vi "SetVariable.vi"(7 "VISA resource name":refnum<visa-resource-name>, 8 "error in (no error)":errorcluster, 9 "Vaste käsk":string="E", 10 "Sisu":string, 11 "Käsk":string="F") -> (3 "Väljund":string)   [LabVIEW 2012]
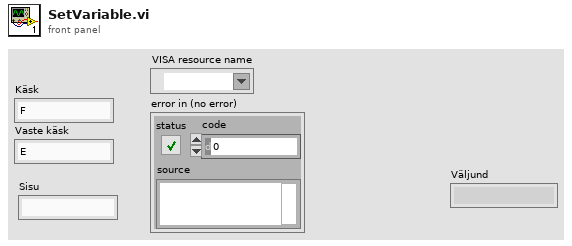
[diagram p1: front panel]
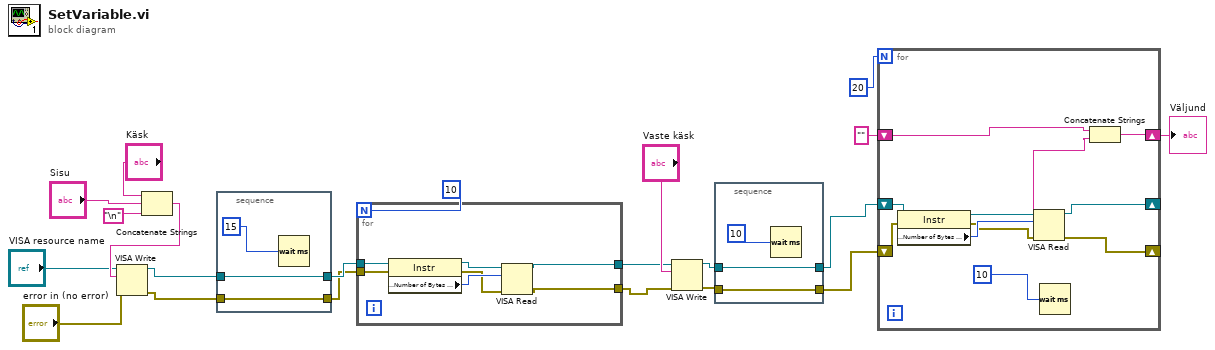
[diagram p0: block diagram]
diagram:
  n1 = Concatenate Strings("Käsk", "Sisu", "\n") -> (w16:string)
  n2 = VISA Write(VISA resource name="VISA resource name", write buffer=w16, error in (no error)="error in (no error)") -> (VISA resource name out=w21:refnum<visa-resource-name>, error out=w20:errorcluster)  [unwired: 1 out]
  n3 = stacked-sequence {
    tunnel: w20 -> [w24]
    tunnel: [w24] -> w18
    tunnel: w21 -> [w23]
    tunnel: [w23] -> w19
    frame #0 {
      n4 = Wait (ms)(milliseconds to wait=u32 15 ("delay Command")) -> ()  [unwired: 1 out]
    }
  }
  n5 = for {
    N: 10 -> [_]
    tunnel: w19 -> [w31]
    tunnel: w18 -> [w30]
    tunnel: [w26] -> w9
    tunnel: [w25] -> w8
    n6 = property class="Instr"(reference=w31, error in=w30) -> (reference out=w29:refnum<visa-resource-name>, error out=w27:errorcluster, "Serial Settings:Number of Bytes at Serial Port"=w28:u32)
    n7 = VISA Read(VISA resource name=w29, byte count=w28, error in (no error)=w27) -> (VISA resource name out=w26:refnum<visa-resource-name>, error out=w25:errorcluster)  [unwired: 2 out]
  }
  n8 = VISA Write(VISA resource name=w9, write buffer="Vaste käsk", error in (no error)=w8) -> (VISA resource name out=w11:refnum<visa-resource-name>, error out=w10:errorcluster)  [unwired: 1 out]
  n9 = stacked-sequence {
    tunnel: w10 -> [w34]
    tunnel: [w34] -> w7
    tunnel: w11 -> [w33]
    tunnel: [w33] -> w6
    frame #0 {
      n10 = Wait (ms)(milliseconds to wait=u32 10 ("delay Input")) -> ()  [unwired: 1 out]
    }
  }
  n11 = for {
    N: 20 -> [_]
    shift-right: [w35] -> w3
    shift-left: "" -> [w36]
    shift-right: [w40] -> _
    shift-left: w6 -> [w38]
    shift-right: [w39] -> _
    shift-left: w7 -> [w41]
    n12 = property class="Instr"(reference=w38, error in=w41) -> (reference out=w45:refnum<visa-resource-name>, error out=w43:errorcluster, "Serial Settings:Number of Bytes at Serial Port"=w44:u32)
    n13 = VISA Read(VISA resource name=w45, byte count=w44, error in (no error)=w43) -> (VISA resource name out=w40:refnum<visa-resource-name>, read buffer=w37:string, error out=w39:errorcluster)  [unwired: 1 out]
    n14 = Wait (ms)(milliseconds to wait=u32 10 ("delay Input 2")) -> ()  [unwired: 1 out]
    n15 = Concatenate Strings(w36, w37) -> (w35:string)
  }
  "Väljund" <- w3
